vi "String to DBL.vi"(8 "error in":errorcluster, 11 "Integer String":string) -> (0 "error out":errorcluster, 3 "DBL":dbl)   [LabVIEW 2019, in "Electronic Datasheet.lvlib"]
doc: "Converts the string representation of a number in a specified base to an equivalent 32-bit signed integer."
uses:
  Core/Electronic Datasheet.lvlib
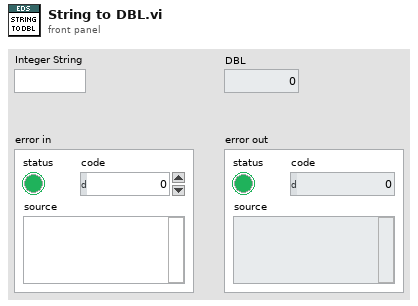
[diagram p1: front panel]
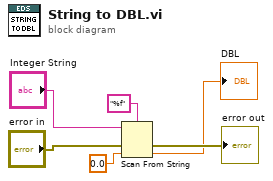
[diagram p0: block diagram]
diagram:
  n1 = Scan From String(format string="%f", input string="Integer String", error in="error in", default 1=0.0) -> (error out=→"error out":errorcluster, output 1=→"DBL":dbl)  [unwired: 1 in, 2 out]
